vi "XControl with User Events Init.vi"(3 "Container State":T3, 4 "Previous State":variant, 5 "Previous Version":T2) -> (2 "Current State":T1)   [LabVIEW 2009, in "XControlUserEvents.xctl"]
doc: "Demonstration of an XControl.\n\nAAL 9/09"
uses:
  XControlUserEvents.xctl
  XControl with User Events State.ctl
  <vilib>/_xctls/Container State.ctl
  <vilib>/_xctls/Version.ctl
  <vilib>/_xctls/XControlSupport.lvlib
panel:
  in  "Default Indicator State":T1
  in  "Default Control State":T1
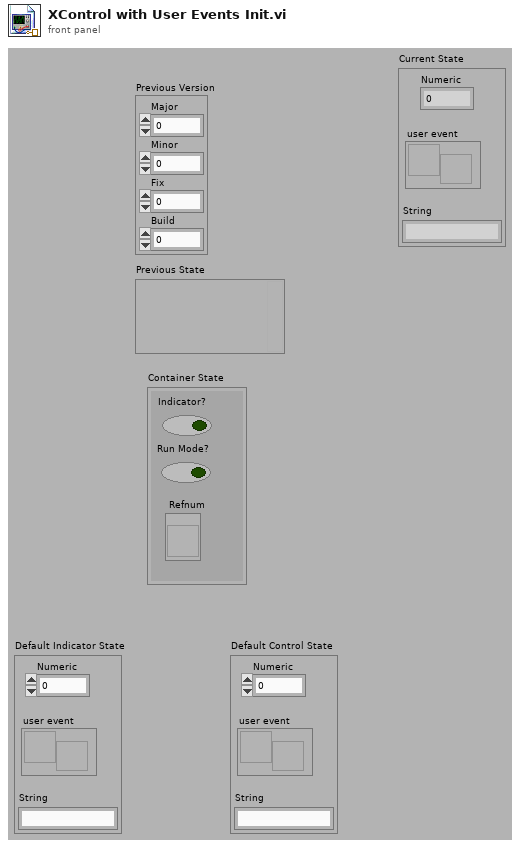
[diagram p1: front panel]
types:
  T1 = typedef "XControlUserEvents.xctl/XControl with User Events State.ctl" = cluster{"Numeric":dbl, "user event":refnum<user-event>, "String":string}
  T2 = typedef "XControlSupport.lvlib/Version.ctl" = cluster{"Major":u16, "Minor":u16, "Fix":u16, "Build":u16}
  T3 = typedef "XControlSupport.lvlib/Container State.ctl" = cluster{"Indicator?":bool, "Run Mode?":bool, " Refnum":refnum<vi>}
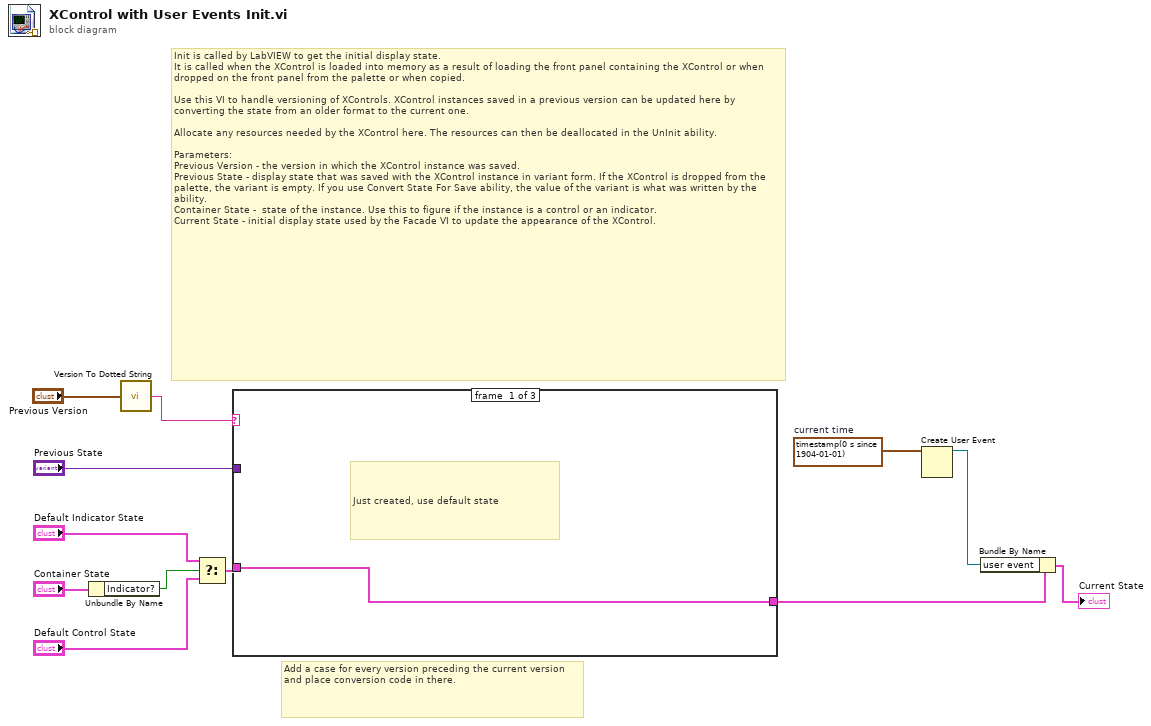
[diagram p0: block diagram]
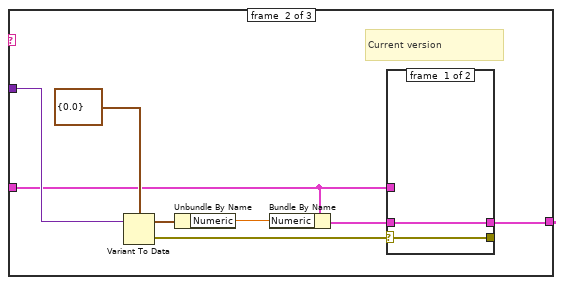
[diagram p2: hidden frame]
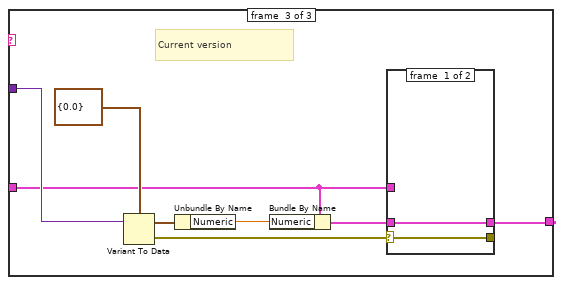
[diagram p4: hidden frame]
diagram:
  w3 = timestamp(0 s since 1904-01-01)  # current time
  # "Add a case for every version preceding the current version and place conversion code in there."
  # "Init is called by LabVIEW to get the initial display state.\nIt is called when the XControl is loaded into memory as a result of loading the front panel containing the XControl or when dropped on the front panel from the palette or when copied.\n\nUse this VI to handle versioning of XControls. XControl instances saved in a previous version can be updated here by converting the state from an older format to the current one.\n\nAllocate any resources needed by the XControl here. The resources can then be deallocated in the UnInit ability.\n\nParameters:\nPrevious Version - the version in which the XControl instance was saved.\nPrevious State - display state that was saved with the XControl instance in variant form. If the XControl is dropped from the palette, the variant is empty. If you use Convert State For Save ability, the value of the variant is what was written by the ability. \nContainer State -  state of the instance. Use this to figure if the instance is a control or an indicator.\nCurrent State - initial display state used by the Facade VI to update the appearance of the XControl."
  n1 = Unbundle By Name("Container State") -> ("Indicator?"=w8:bool)
  n2 = call <vilib>:"Version To Dotted String.vi"("Version"="Previous Version") -> ("String Version"=w5:string)
  n3 = Select(t="Default Indicator State", s=w8, f="Default Control State") -> (s? t:f=w7:T1)
  n4 = case shown="\"1.0.2.0\"" w5 {
    tunnel: "Previous State" -> [_ w21 w33]
    tunnel: [w13 w19 w31] -> w1
    tunnel: w7 -> [w13 w16 w28]
    frame #0 {
      # "Just created, use default state"
    }
    frame #1 {
      # "Current version"
      n5 = Variant To Data(Variant=w21, type=cluster{"Numeric":dbl} {"Numeric"=0.0}) -> (error out=w20:errorcluster, data=w17:cluster{"Numeric":dbl})  [unwired: 1 in]
      n6 = Unbundle By Name(w17) -> ("Numeric"=w15:dbl)
      n7 = Bundle By Name(cluster=w16, "Numeric"=w15) -> (w14:T1)
      n8 = case shown="Error" w20 {
        selector: w20 -> [w23 w24]
        tunnel: w14 -> [w22 _]
        tunnel: [w22 w25] -> w19
        tunnel: w16 -> [_ w25]
        tunnel: [w23 w24] -> _
        frame #0 {
        }
        frame #1 {
          # "Error converting previously \nsaved state. Use default instead."
        }
      }
    }
    frame #2 {
      # "Current version"
      n9 = Variant To Data(Variant=w33, type=cluster{"Numeric":dbl} {"Numeric"=0.0}) -> (error out=w32:errorcluster, data=w29:cluster{"Numeric":dbl})  [unwired: 1 in]
      n10 = Unbundle By Name(w29) -> ("Numeric"=w27:dbl)
      n11 = Bundle By Name(cluster=w28, "Numeric"=w27) -> (w26:T1)
      n12 = case shown="Error" w32 {
        selector: w32 -> [w35 w36]
        tunnel: w26 -> [w34 _]
        tunnel: [w34 w37] -> w31
        tunnel: w28 -> [_ w37]
        tunnel: [w35 w36] -> _
        frame #0 {
        }
        frame #1 {
          # "Error converting previously \nsaved state. Use default instead."
        }
      }
    }
  }
  n13 = Create User Event(user event datatype=w3) -> (user event=w4:refnum<user-event>)  [unwired: 1 in, 1 out]
  n14 = Bundle By Name(cluster=w1, "user event"=w4) -> (→"Current State":T1)
